vi "Generate Simulated AI.vi"(8 "error in (no error)":errorcluster, 9 "Sampling_Config":T2={"Fs"=1000.0, "#s"=1000.0} {"Fs" format="%.2p"}, 10 "Signal_Config":T1={"offset"=0.0, "frequency"=10.0, "amplitude"=1.0} {"amplitude" format="%#_13g"; "frequency" format="%#_13g"; "offset" format="%0.2p"}, 11 "Signal Type":T3) -> (0 "error out":errorcluster, 3 "Graph Data":waveform(dbl))   [LabVIEW 2023, in "Analog Signal.lvclass"]
uses:
  Analog Signal.lvclass
  Signal Type.ctl
  Analog Signal.lvclass/Analog Signal.ctl
  <vilib>/measure/NI_MABase.lvlib
  Signal Config.ctl
  Sampling Config.ctl
panel:
  # "Connector Pane"
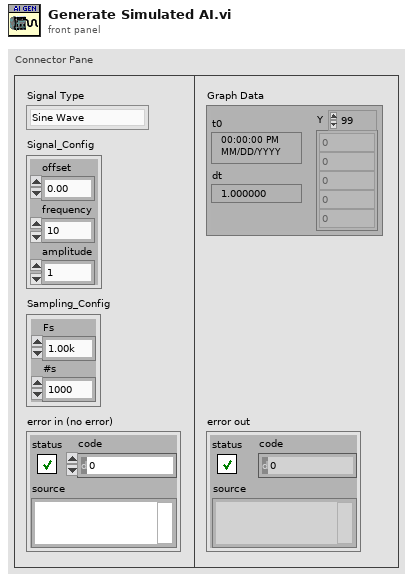
[diagram p1: front panel]
types:
  T1 = typedef "Analog Signal.lvclass/Signal Config.ctl" = cluster{"offset":dbl, "frequency":dbl, "amplitude":dbl}
  T2 = typedef "Analog Signal.lvclass/Sampling Config.ctl" = cluster{"Fs":dbl, "#s":dbl}
  T3 = typedef "Analog Signal.lvclass/Signal Type.ctl" = enum16{"Sine Wave", "Square Wave"}
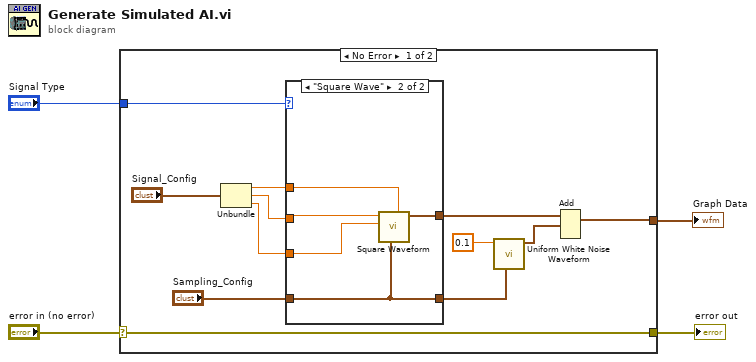
[diagram p0: block diagram]
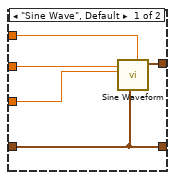
[diagram p2: hidden frame]
diagram:
  n1 = case shown="No Error" "error in (no error)" {
    selector: "error in (no error)" -> [w16 w27]
    tunnel: [w16 w27] -> w3
    tunnel: [w5 _] -> w1
    tunnel: "Signal Type" -> [w15 _]
    frame No Error {
      n2 = Unbundle("Signal_Config") -> ("offset"=w12:dbl, "frequency"=w11:dbl, "amplitude"=w10:dbl)
      n3 = case shown="\"Square Wave\"" w15 {
        tunnel: [w21 w26] -> w7
        tunnel: w11 -> [w20 w24]
        tunnel: w10 -> [w19 w23]
        tunnel: w12 -> [w18 w25]
        tunnel: "Sampling_Config" -> [w17 w22]
        tunnel: [w17 w22] -> w9
        frame "Sine Wave", Default {
          n4 = call <vilib>:"Sine Waveform.vi"("offset"=w18, "sampling info"=w17, "amplitude"=w19, "frequency"=w20) -> ("signal out"=w21:waveform(dbl))  [unwired: 6 in, 1 out]
        }
        frame "Square Wave" {
          n5 = call <vilib>:"Square Waveform.vi"("offset"=w25, "sampling info"=w22, "amplitude"=w23, "frequency"=w24) -> ("signal out"=w26:waveform(dbl))  [unwired: 6 in, 1 out]
        }
      }
      n6 = call <vilib>:"Uniform White Noise Waveform.vi"("sampling info"=w9, "amplitude"=0.1 ("noise (rms)")) -> ("signal out"=w6:waveform(dbl))  [unwired: 8 in, 1 out]
      n7 = Add(1:w6, 2:w7) -> (0:w5:waveform(dbl))  [unwired: 1 in, 1 out]
    }
    frame Error {
    }
  }
  "error out" <- w3
  "Graph Data" <- w1
